vi "Live 3-camera test.vi"(8 "Gain":i32=100 min=100 max=2000 step=1, 9 "Exposure time (ms)":dbl=100.0 min=1.0 max=10000.0 step=1.0) -> (2 "Image out":T1(plugin-control))   [LabVIEW 2017]
panel:
  in  "Camera":u16(ring) items=["Red", "Green", "Blue"]
  in  "stop":bool
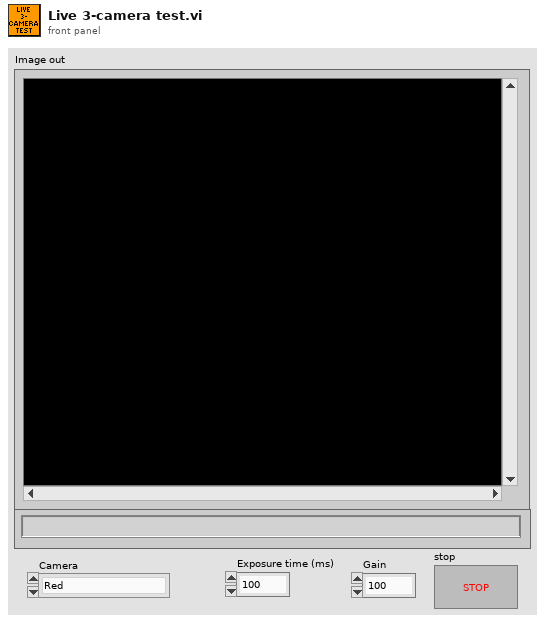
[diagram p1: front panel]
types:
  T1 = typedef "IMAQ Image.ctl" = refnum<image>
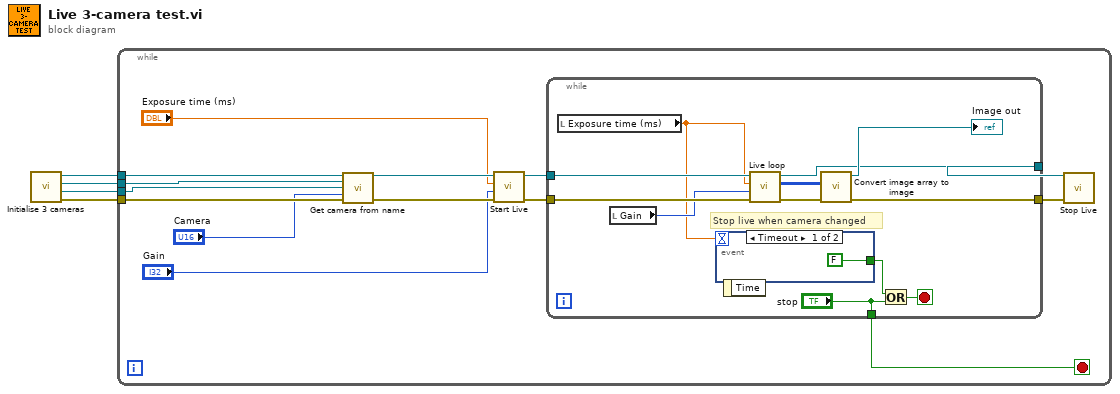
[diagram p0: block diagram]
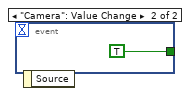
[diagram p2: hidden frame]
diagram:
  n1 = call "Initialise 3 cameras.vi"() -> ("Error Out"=w3:errorcluster, "Blue camera ref"=w1:refnum<k24>, "Green camera ref"=w2:refnum<k24>, "Red camera ref"=w4:refnum<k24>)  [unwired: 8 in]
  n2 = while {
    tunnel: w4 -> [w16]
    tunnel: w3 -> [w13]
    tunnel: w2 -> [w15]
    tunnel: w1 -> [w14]
    stop <- w5 stop-if-true
    n3 = call "Get camera from name.vi"("Red ref"=w16, "Green ref"=w15, "Blue ref"=w14, "Camera"="Camera", "Error In"=w13) -> ("Camera reference out"=w17:refnum<k24>, "Error Out"=w18:errorcluster)  [unwired: 9 in]
    n4 = call "Start Live.vi"("Error In"=w18, "Gain in"="Gain", "Exposure time (ms)"="Exposure time (ms)", "Camera reference in"=w17) -> ("Error Out"=w9:errorcluster, "Camera reference out"=w8:refnum<k24>)  [unwired: 5 in]
    n5 = while {
      tunnel: w8 -> [w30]
      tunnel: w9 -> [w29]
      tunnel: [w24] -> w7
      tunnel: [w23] -> w6
      tunnel: ["stop"] -> w5
      stop <- w21 stop-if-true
      # "Stop live when camera changed"
      n6 = local read "Exposure time (ms)"() -> (w19:dbl)
      n7 = local read "Gain"() -> (w28:i32)
      n8 = event shown="[0] Timeout" {
        selector: _ -> [_ _]
        dyn-events: _ -> [_ _]
        timeout: w19 -> [_ _]
        tunnel: [FALSE TRUE] -> w22
        event Timeout {
          n9 = event-data() -> ()  [unwired: 1 in, 1 out]
        }
        event "Camera": Value Change {
          n10 = event-data() -> ()  [unwired: 1 in, 1 out]
        }
      }
      n11 = call "Live loop.vi"("Error In"=w29, "Gain"=w28, "Exposure time (ms)"=w19, "Camera reference in"=w30) -> ("Error Out"=w26:errorcluster, "Image Array"=w27:u16[][], "Camera reference out"=w24:refnum<k24>)  [unwired: 4 in]
      n12 = call "Convert image array to image.vi"("Error In"=w26, "Array"=w27) -> ("error out"=w23:errorcluster, "Image Out"=→"Image out":T1)  [unwired: 7 in]
      n13 = Or(x=w22, y="stop") -> (x .or. y?=w21:bool)
    }
    n14 = call "Stop Live.vi"("Camera reference in"=w7, "Error In"=w6) -> ()  [unwired: 16 in, 2 out]
  }
